vi "testStopServersAandB.vi"(8 "error in (no error)":errorcluster) -> (0 "error out":errorcluster)   [LabVIEW 2018]
uses:
  src/TcpServer/TcpServer.lvclass
  src/TcpServer/TcpServer.lvclass/TcpServer.ctl
  <vilib>/addons/_JKI Toolkits/Caraya/classes/Assert/Assert Equal Value_Variant.vi
  src/TcpServerCmd/TcpServerCmd.lvclass
  src/TcpServerTel/TcpServerTel.lvclass
  <vilib>/addons/_JKI Toolkits/Caraya/classes/Test/Test.lvclass
  <vilib>/addons/_JKI Toolkits/Caraya/classes/Assert/Assert.lvclass
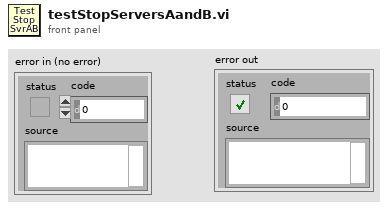
[diagram p1: front panel]
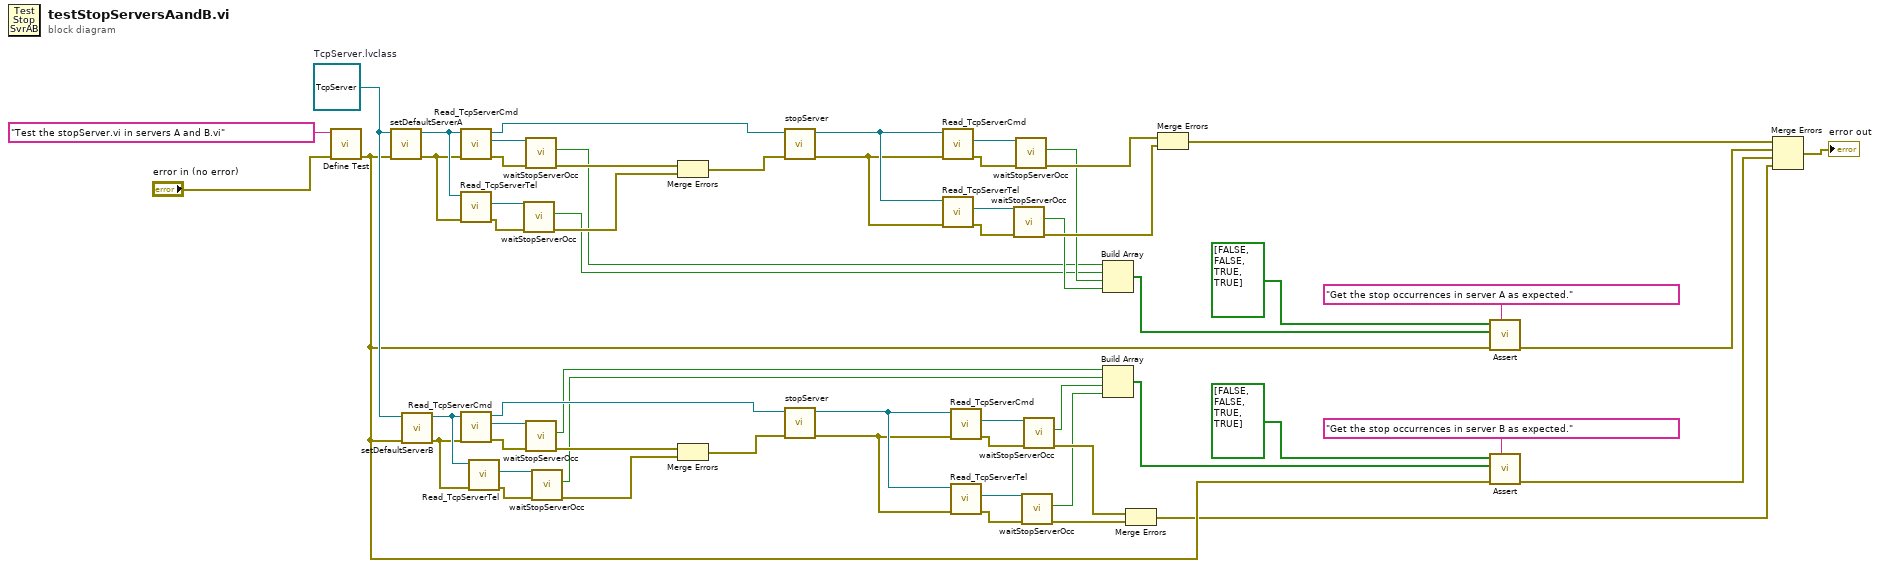
[diagram p0: block diagram]
diagram:
  w39 = refnum<class "TcpServer.lvclass"> refnum  # TcpServer.lvclass
  n1 = call <vilib>:"Define Test.vi"("error in (no error)"="error in (no error)", "Label (VI Title)"="Test the stopServer.vi in servers A and B.vi") -> ("error out"=w8:errorcluster)  [unwired: 9 in]
  n2 = call "setDefaultServerA.vi"("error in (no error)"=w8, "TcpServer.lvclass"=w39) -> ("error out"=w40:errorcluster, "tcpServer out"=w41:refnum<class "TcpServer.lvclass">)  [unwired: 8 in]
  n3 = call "setDefaultServerB.vi"("error in (no error)"=w8, "TcpServer.lvclass"=w39) -> ("error out"=w17:errorcluster, "tcpServer out"=w18:refnum<class "TcpServer.lvclass">)  [unwired: 8 in]
  n4 = call "Read_TcpServerCmd.vi"("error in (no error)"=w40, "TcpServer in"=w41) -> ("error out"=w54:errorcluster, "TcpServerCmd.lvclass"=w55:refnum<class "TcpServerCmd.lvclass">, "TcpServer out"=w57:refnum<class "TcpServer.lvclass">)  [unwired: 7 in]
  n5 = call "Read_TcpServerTel.vi"("error in (no error)"=w40, "TcpServer in"=w41) -> ("error out"=w52:errorcluster, "TcpServerTel.lvclass"=w53:refnum<class "TcpServerTel.lvclass">)  [unwired: 7 in, 1 out]
  n6 = call "Read_TcpServerCmd.vi"("error in (no error)"=w17, "TcpServer in"=w18) -> ("error out"=w28:errorcluster, "TcpServerCmd.lvclass"=w27:refnum<class "TcpServerCmd.lvclass">, "TcpServer out"=w25:refnum<class "TcpServer.lvclass">)  [unwired: 7 in]
  n7 = call "Read_TcpServerTel.vi"("error in (no error)"=w17, "TcpServer in"=w18) -> ("error out"=w20:errorcluster, "TcpServerTel.lvclass"=w19:refnum<class "TcpServerTel.lvclass">)  [unwired: 7 in, 1 out]
  n8 = call "waitStopServerOcc.vi"("error in (no error)"=w52, "TcpServerTel in"=w53) -> ("error out"=w51:errorcluster, "stopServer"=w13:bool)  [unwired: 7 in, 1 out]
  n9 = call "waitStopServerOcc.vi"("error in (no error)"=w54, "TcpServerCmd in"=w55) -> ("error out"=w50:errorcluster, "stopServer"=w14:bool)  [unwired: 7 in, 1 out]
  n10 = call "waitStopServerOcc.vi"("error in (no error)"=w28, "TcpServerCmd in"=w27) -> ("error out"=w29:errorcluster, "stopServer"=w7:bool)  [unwired: 7 in, 1 out]
  n11 = call "waitStopServerOcc.vi"("error in (no error)"=w20, "TcpServerTel in"=w19) -> ("error out"=w21:errorcluster, "stopServer"=w6:bool)  [unwired: 7 in, 1 out]
  n12 = Merge Errors(w50, w51) -> (w56:errorcluster)
  n13 = Merge Errors(w29, w21) -> (w26:errorcluster)
  n14 = call "stopServer.vi"("error in (no error)"=w56, "tcpServer in"=w57) -> ("error out"=w46:errorcluster, "tcpServer out"=w47:refnum<class "TcpServer.lvclass">)  [unwired: 8 in]
  n15 = call "stopServer.vi"("error in (no error)"=w26, "tcpServer in"=w25) -> ("error out"=w15:errorcluster, "tcpServer out"=w16:refnum<class "TcpServer.lvclass">)  [unwired: 8 in]
  n16 = call "Read_TcpServerCmd.vi"("error in (no error)"=w46, "TcpServer in"=w47) -> ("error out"=w44:errorcluster, "TcpServerCmd.lvclass"=w45:refnum<class "TcpServerCmd.lvclass">)  [unwired: 7 in, 1 out]
  n17 = call "Read_TcpServerTel.vi"("error in (no error)"=w46, "TcpServer in"=w47) -> ("error out"=w42:errorcluster, "TcpServerTel.lvclass"=w43:refnum<class "TcpServerTel.lvclass">)  [unwired: 7 in, 1 out]
  n18 = call "Read_TcpServerCmd.vi"("error in (no error)"=w15, "TcpServer in"=w16) -> ("error out"=w32:errorcluster, "TcpServerCmd.lvclass"=w31:refnum<class "TcpServerCmd.lvclass">)  [unwired: 7 in, 1 out]
  n19 = call "Read_TcpServerTel.vi"("error in (no error)"=w15, "TcpServer in"=w16) -> ("error out"=w24:errorcluster, "TcpServerTel.lvclass"=w23:refnum<class "TcpServerTel.lvclass">)  [unwired: 7 in, 1 out]
  n20 = call "waitStopServerOcc.vi"("error in (no error)"=w42, "TcpServerTel in"=w43) -> ("error out"=w48:errorcluster, "stopServer"=w35:bool)  [unwired: 7 in, 1 out]
  n21 = call "waitStopServerOcc.vi"("error in (no error)"=w44, "TcpServerCmd in"=w45) -> ("error out"=w49:errorcluster, "stopServer"=w36:bool)  [unwired: 7 in, 1 out]
  n22 = call "waitStopServerOcc.vi"("error in (no error)"=w24, "TcpServerTel in"=w23) -> ("error out"=w22:errorcluster, "stopServer"=w4:bool)  [unwired: 7 in, 1 out]
  n23 = call "waitStopServerOcc.vi"("error in (no error)"=w32, "TcpServerCmd in"=w31) -> ("error out"=w30:errorcluster, "stopServer"=w5:bool)  [unwired: 7 in, 1 out]
  n24 = Build Array(w14, w13, w36, w35) -> (w12:bool[])
  n25 = Build Array(w7, w6, w5, w4) -> (w3:bool[])
  n26 = Merge Errors(w30, w22) -> (w1:errorcluster)
  n27 = Merge Errors(w49, w48) -> (w37:errorcluster)
  n28 = call-poly <vilib>:"Assert.vi"("Label"="Get the stop occurrences in server A as expected.", "error in (no error)"=w8, "Y"=w12, "X"=bool[] [FALSE, FALSE, TRUE, TRUE]) -> ("error out"=w33:errorcluster)  [unwired: 7 in]
  n29 = call-poly <vilib>:"Assert.vi"("Label"="Get the stop occurrences in server B as expected.", "error in (no error)"=w8, "Y"=w3, "X"=bool[] [FALSE, FALSE, TRUE, TRUE]) -> ("error out"=w2:errorcluster)  [unwired: 7 in]
  n30 = Merge Errors(w37, w33, w2, w1) -> (→"error out":errorcluster)
